vi "UTILITY Delete Empty String Cells 2D.vi"(11 "Array with Empty Cells":string[][](array[string])) -> (3 "Array w/o Empty Cells":string[][](array[string]))   [LabVIEW 2016]
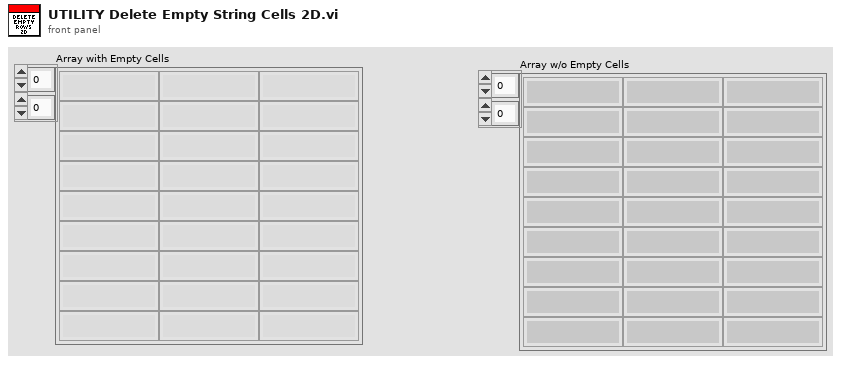
[diagram p1: front panel]
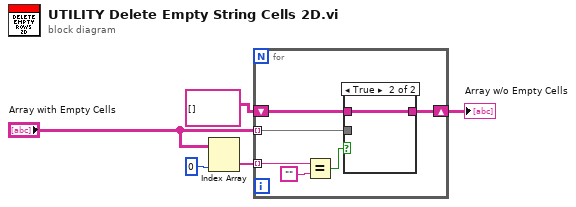
[diagram p0: block diagram]
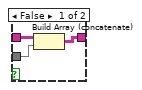
[diagram p2: hidden frame]
diagram:
  n1 = Index Array(array="Array with Empty Cells", index (col)=0 ("disabled index (col)")) -> (element=w1:string[])  [unwired: 1 in]
  n2 = for {
    tunnel: "Array with Empty Cells" -> [w8] mode=indexing
    shift-right: [w7] -> w5
    shift-left: string[][] [] -> [w9]
    tunnel: w1 -> [w6] mode=indexing
    n3 = Equal?(x=w6, y="") -> (x = y?=w10:bool)
    n4 = case shown="True" w10 {
      tunnel: w9 -> [w14 w15]
      tunnel: w8 -> [w13 _]
      tunnel: [w12 w15] -> w7
      frame False {
        n5 = Build Array (concatenate)(w14, w13) -> (w12:string[][])
      }
      frame True {
      }
    }
  }
  "Array w/o Empty Cells" <- w5
